vi "Read Waveform.vi"(8 "error in (no error)":errorcluster, 9 "Source (0: Channel 1)":u16(ring) items=["Channel 1", "Channel 2", "Channel 3", "Channel 4", "Math", "Reference A", "Reference B", "Reference C", "Reference D", "FFT"], 10 "Timeout (10000 ms)":u32=10000, 11 "Tektronic in":refnum<class "Tektronic.lvclass">) -> (0 "error out":errorcluster, 1 "Waveform Data":waveform(dbl)(graph), 3 "Tektronic out":refnum<class "Tektronic.lvclass">)   [LabVIEW 2020, in "Controlador.lvlib" / "Tektronic.lvclass"]
uses:
  Tektronic.lvclass
  C:/Users/scrap/Fork/Modulo_Cloneable_DQMH/Libraries/Controlador/Class/Osciloscope/Osciloscope.lvclass
  Osciloscope/Osciloscope.lvclass/Osciloscope.ctl
  Osciloscope/Read COM.vi
  <instrlib>/Tektronix TDS 200 1000 2000 Series/Public/Data/Read (Single Waveform).vi
  <instrlib>/Tektronix TDS 200 1000 2000 Series/Tektronix TDS 200 1000 2000 Series.lvlib
  Osciloscope/Osciloscope.lvclass
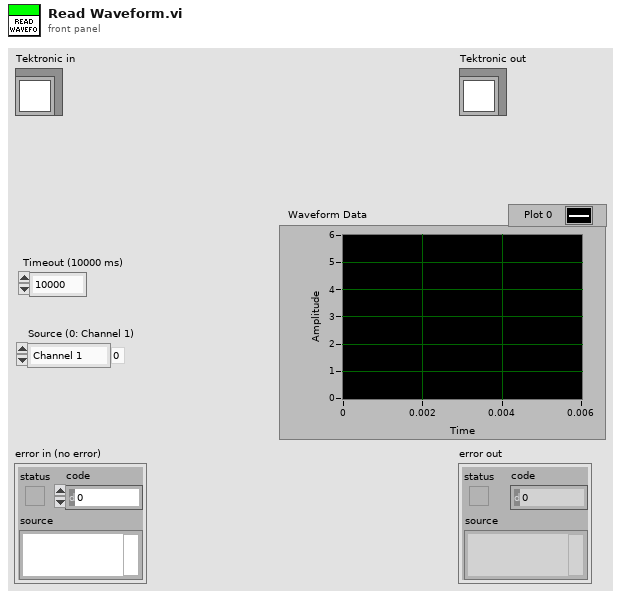
[diagram p1: front panel]
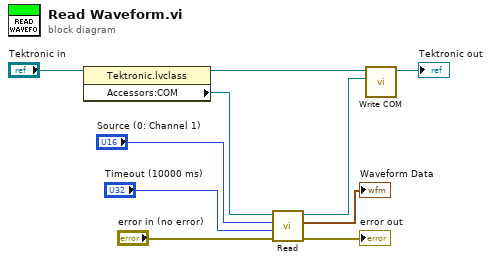
[diagram p0: block diagram]
diagram:
  n1 = property class="Tektronic.lvclass"(reference="Tektronic in") -> (reference out=w3:refnum<class "Tektronic.lvclass">, "Accessors:COM"=w5:refnum<visa-resource-name>)  [unwired: 1 in, 1 out]
  n2 = call-poly <instrlib>:"Read.vi"("error in (no error)"="error in (no error)", "Timeout (10000 ms)"="Timeout (10000 ms)", "Source (0: Channel 1)"="Source (0: Channel 1)", "VISA resource name"=w5) -> ("error out"=→"error out":errorcluster, "Waveform Data"=→"Waveform Data":waveform(dbl), "VISA resource name out"=w4:refnum<visa-resource-name>)  [unwired: 5 in]
  n3 = call "Write COM.vi"("COM"=w4, "Osciloscope in"=w3) -> ("Osciloscope out"=→"Tektronic out":refnum<class "Tektronic.lvclass">)  [unwired: 8 in, 1 out]
